vi "insert_doubles_array.vi"(6 "Time Stamp":timestamp, 8 "error in (no error)":errorcluster, 9 "Values":dbl[](array[numeric]), 10 "paths":string[](array[string]), 11 "Data.PG in":refnum<class "Data.PG.lvclass">) -> (0 "error out":errorcluster, 3 "Data.PG out":refnum<class "Data.PG.lvclass">)   [LabVIEW 2020, in "Data.PG.lvclass"]
uses:
  Data.PG.lvclass
  Data/Typedefs/Operation--enum.ctl
  Data.PG.lvclass/Data.PG.ctl
  <vilib>/JDP Science/PostgreSQL Library/Result/PQ Result.lvclass/PQ Result.ctl
  <vilib>/JDP Science/PostgreSQL Library/Connection/Execute Command (2D string results).vi
  <vilib>/JDP Science/PostgreSQL Library/Result/Clear.vi
  <vilib>/JDP Science/PostgreSQL Library/Connection/Execute Command (Result).vi
  <vilib>/JDP Science/PostgreSQL Library/Connection/Execute (Return first result with rows).vi
  <vilib>/JDP Science/PostgreSQL Library/Connection/Single Command with parameters.vi
  <vilib>/JDP Science/PostgreSQL Library/Result/Get all results as 2D strings array.vi
  <vilib>/JDP Science/PostgreSQL Library/Connection/PQ Connection.lvclass
  Data/Data.lvclass
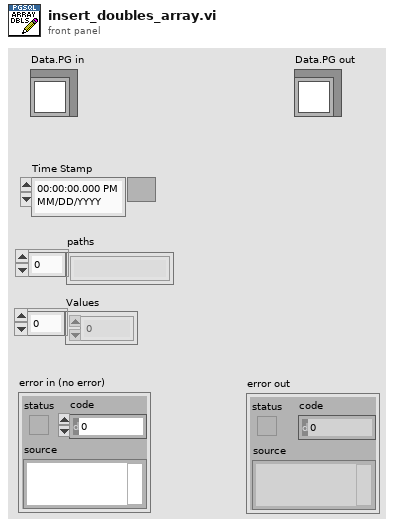
[diagram p1: front panel]
types:
  T1 = typedef "Data.lvclass/Operation--enum.ctl" = enum16{"Read", "Write", "Write + Append"}
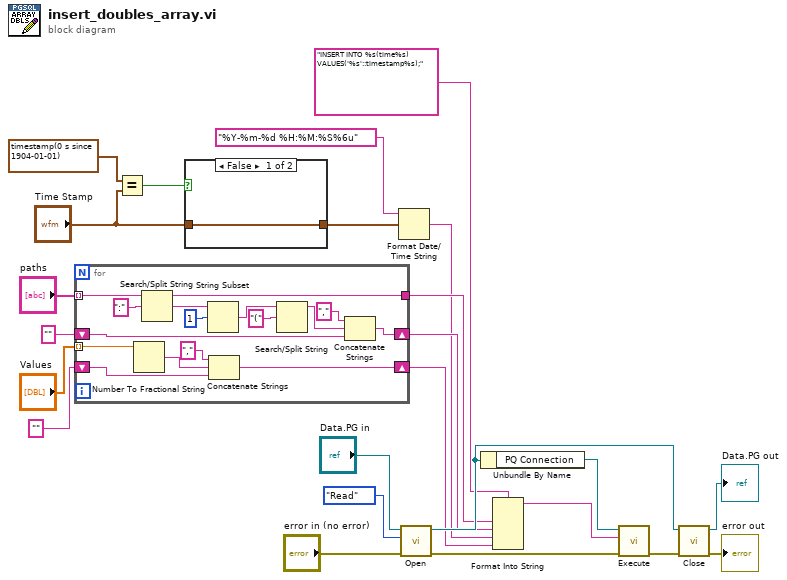
[diagram p0: block diagram]
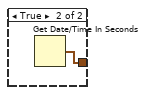
[diagram p2: hidden frame]
diagram:
  n1 = for {
    tunnel: "paths" -> [w37] mode=indexing
    tunnel: "Values" -> [w32] mode=indexing
    shift-right: [w36] -> w9
    shift-left: "" -> [w35]
    tunnel: [w34] -> w10
    shift-right: [w29] -> w6
    shift-left: "" -> [w28]
    n2 = Number To Fractional String(number=w32) -> (F-format string=w31:string)  [unwired: 3 in]
    n3 = Search/Split String(string=w37, search string/char (-)=":") -> (substring before match=w34:string, match + rest of string=w39:string)  [unwired: 1 in, 1 out]
    n4 = String Subset(string=w39, offset (0)=1) -> (substring=w27:string)  [unwired: 1 in]
    n5 = Concatenate Strings("," ("string"), w31, w28) -> (w29:string)
    n6 = Search/Split String(string=w27, search string/char (-)="(") -> (substring before match=w26:string)  [unwired: 1 in, 2 out]
    n7 = Concatenate Strings("," ("string"), w26, w35) -> (w36:string)
  }
  n8 = Equal?(x=timestamp(0 s since 1904-01-01), y="Time Stamp") -> (x = y?=w3:bool)
  n9 = case shown="False" w3 {
    tunnel: [w41 w42] -> w4
    tunnel: "Time Stamp" -> [w41 _]
    frame False {
    }
    frame True {
      n10 = Get Date/Time In Seconds() -> (seconds since 1Jan1904=w42:timestamp)
    }
  }
  n11 = Format Date/Time String(time format string (%c)="%Y-%m-%d %H:%M:%S%6u", seconds (now)=w4) -> (date/time string=w8:string)  [unwired: 1 in]
  n12 = call-dynamic "Open.vi"("error in (no error)"="error in (no error)", "Operation"=Operation--enum."Read", "Data.PG in"="Data.PG in") -> ("error out"=w21:errorcluster, "Data.PG out"=w16:refnum<class "Data.PG.lvclass">)  [unwired: 7 in]
  n13 = Unbundle By Name(w16) -> ("PQ Connection"=w15:refnum<class "PQ Connection.lvclass">)
  n14 = Format Into String(format string="INSERT INTO %s(time%s) VALUES('%s'::timestamp%s);", w10, w9, w8, w6) -> (resulting string=w17:string)  [unwired: 2 in, 1 out]
  n15 = call-poly <vilib>:"Execute.vi"("error in (no error)"=w21, "SQL"=w17, "PQ Connection in"=w15) -> ("error out"=w20:errorcluster)  [unwired: 5 in, 3 out]
  n16 = call-dynamic "Close.vi"("error in (no error)"=w20, "Data.PG in"=w16) -> ("error out"=→"error out":errorcluster, "Data.PG out"=→"Data.PG out":refnum<class "Data.PG.lvclass">)  [unwired: 8 in]
